vi "Watch Project.vi"(8 "error in (no error)":errorcluster, 10 "Project Path":path, 11 "WebProjectWatcher in":refnum<class "WebProjectWatcher.lvclass">) -> (0 "error out":errorcluster, 3 "WebProjectWatcher out":refnum<class "WebProjectWatcher.lvclass">)   [LabVIEW 2020, in "PicoG-Processor.lvlib" / "WebProjectWatcher.lvclass"]
uses:
  WebProjectWatcher.lvclass
  WebProjectWatcher.lvclass/WebProjectWatcher.ctl
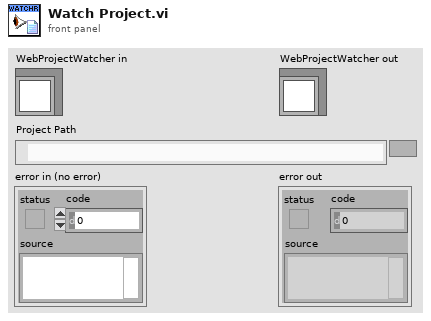
[diagram p1: front panel]
types:
  T1 = typedef "PicoG-Processor.lvlib/WebProjectWatcher.lvclass/Ref Data.ctl" = cluster{"Builds Callbacks":T2[], "Project Path":path, "Close":bool}
  T2 = typedef "PicoG-Processor.lvlib/WebProjectWatcher.lvclass/Builds Callback.ctl" = cluster{"Callback":refnum<vi>, "Owner":refnum<class>}
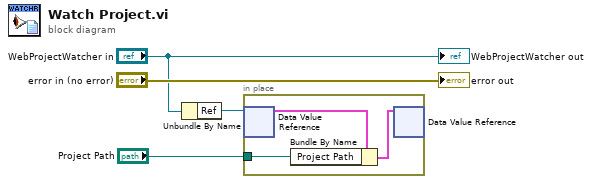
[diagram p0: block diagram]
diagram:
  n1 = Unbundle By Name("WebProjectWatcher in") -> ("Ref"=w3:refnum<data-value>)
  n2 = in-place {
    in-place-border: "Project Path" -> [w5]
    n3 = in-place-dvr #1(w3) -> (w7:T1)  [unwired: 1 out]
    n4 = Bundle By Name(cluster=w7, "Project Path"=w5) -> (w6:T1)
    n5 = in-place-dvr #1(w6) -> ()  [unwired: 2 out]
  }
  "error out" <- "error in (no error)"
  "WebProjectWatcher out" <- "WebProjectWatcher in"
